vi "PosCentersBackAreaQuadrada.vi"(8 "Robô fora?":bool=TRUE, 9 "geometry":T1, 10 "Defensores":u32[](array[numeric]), 11 "Pos Bola":dbl[](array[numeric]) format="%#_13g") -> (2 "Pos Centers Back":dbl[][](array[numeric]), 3 "Central Position":dbl[](array[numeric]))   [LabVIEW 2017]
uses:
  Core/Field Size.ctl
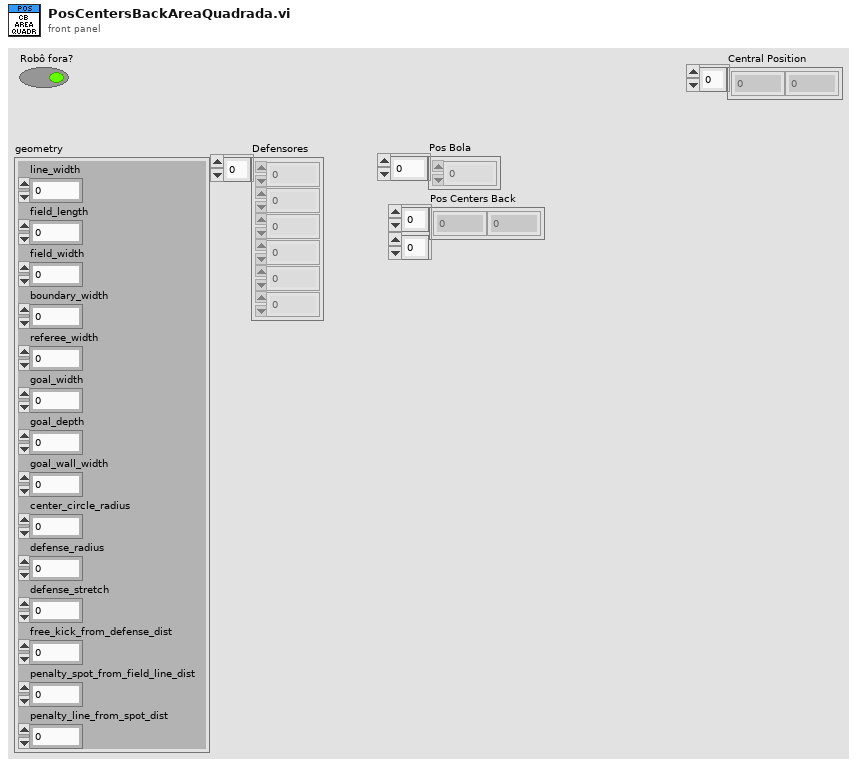
[diagram p1: front panel]
types:
  T1 = typedef "Field Size.ctl" = cluster{"line_width":u32, "field_length":u32, "field_width":u32, "boundary_width":u32, "referee_width":u32, "goal_width":u32, "goal_depth":u32, "goal_wall_width":u32, "center_circle_radius":u32, "defense_radius":u32, "defense_stretch":u32, "free_kick_from_defense_dist":u32, "penalty_spot_from_field_line_dist":u32, "penalty_line_from_spot_dist":u32}
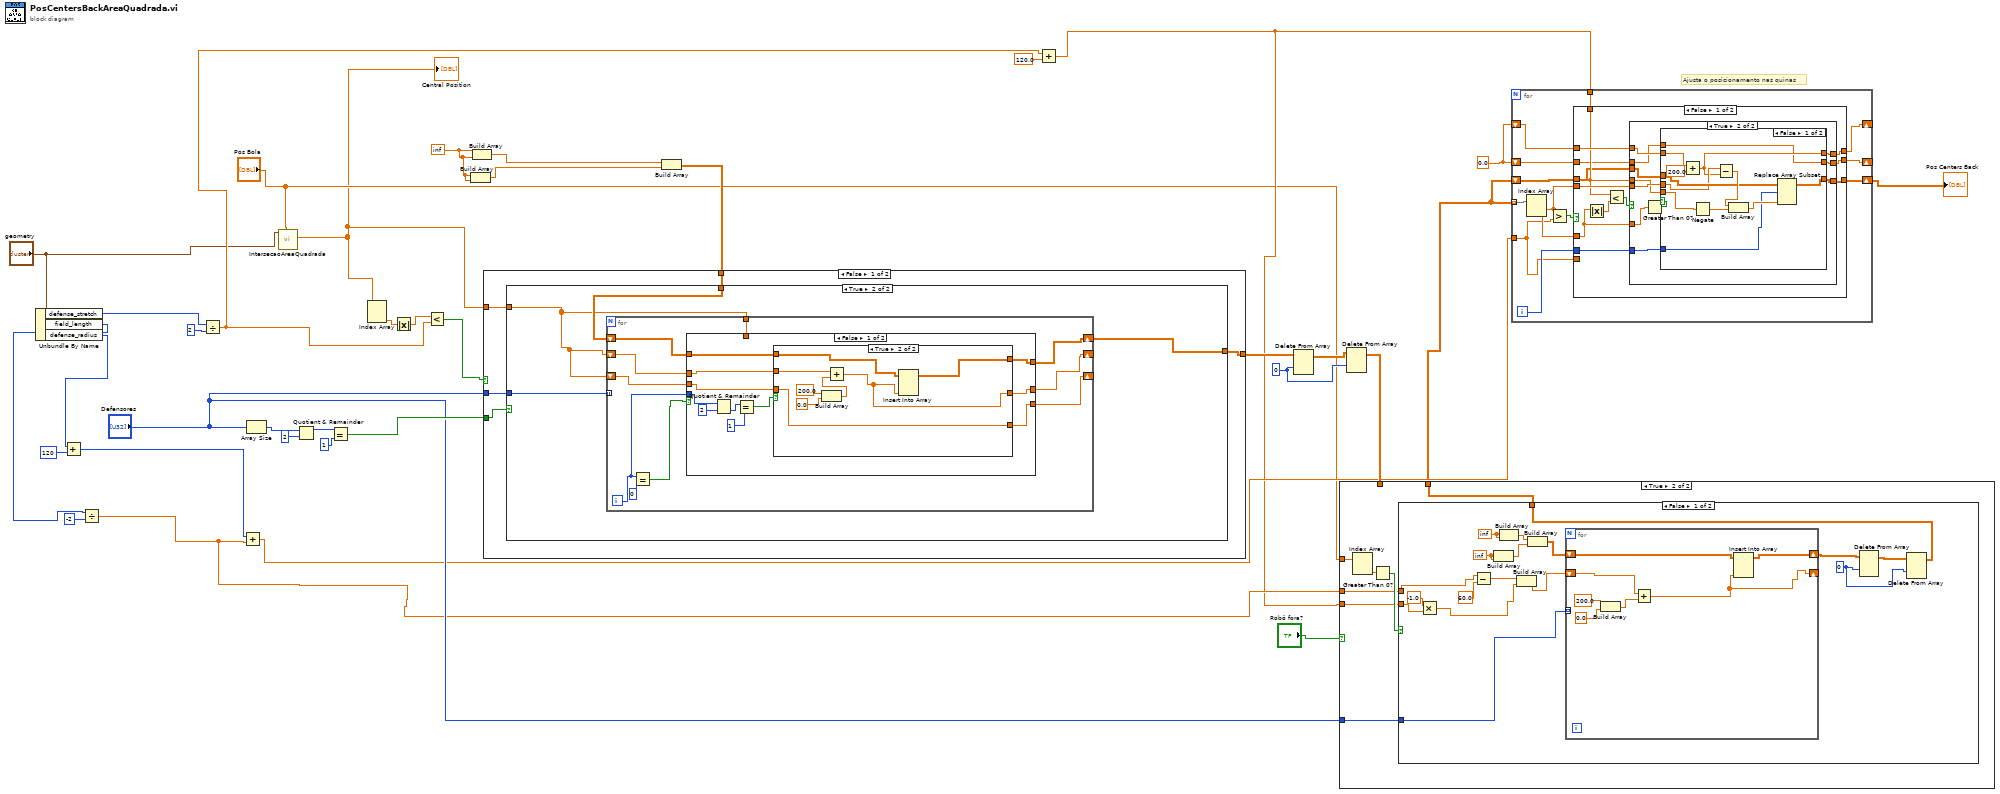
[diagram p0: block diagram]
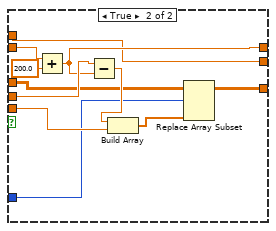
[diagram p3: hidden frame]
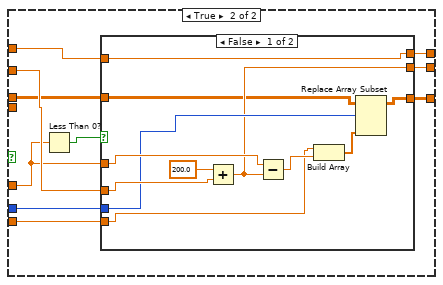
[diagram p4: hidden frame]
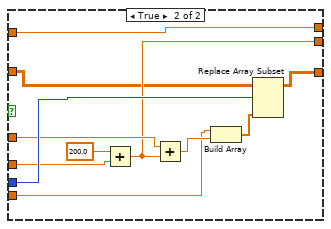
[diagram p5: hidden frame]
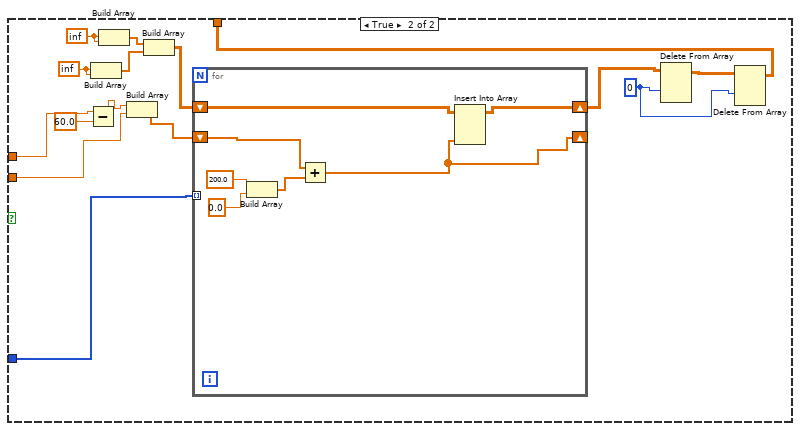
[diagram p7: hidden frame]
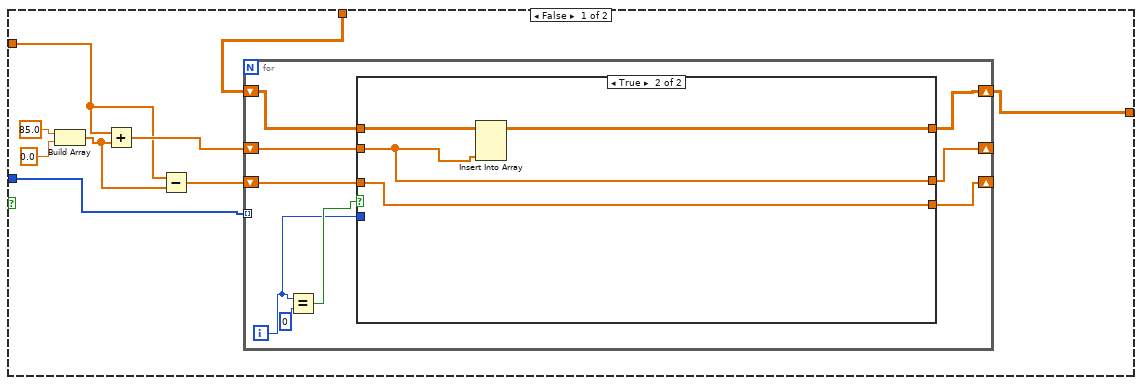
[diagram p8: hidden frame]
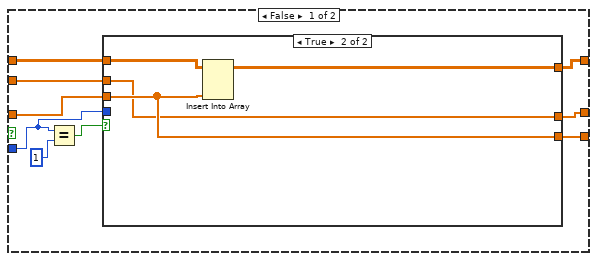
[diagram p9: hidden frame]
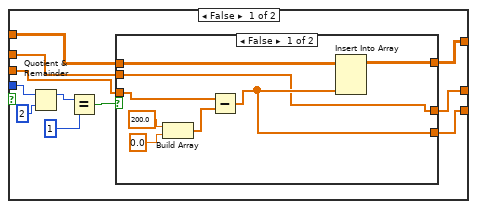
[diagram p10: hidden frame]
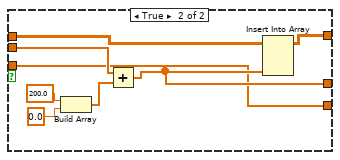
[diagram p11: hidden frame]
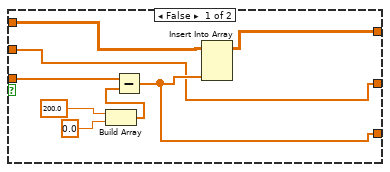
[diagram p12: hidden frame]
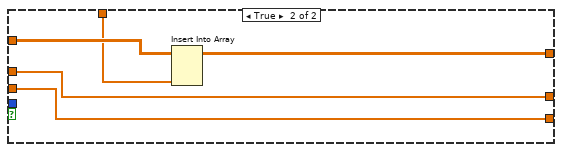
[diagram p13: hidden frame]
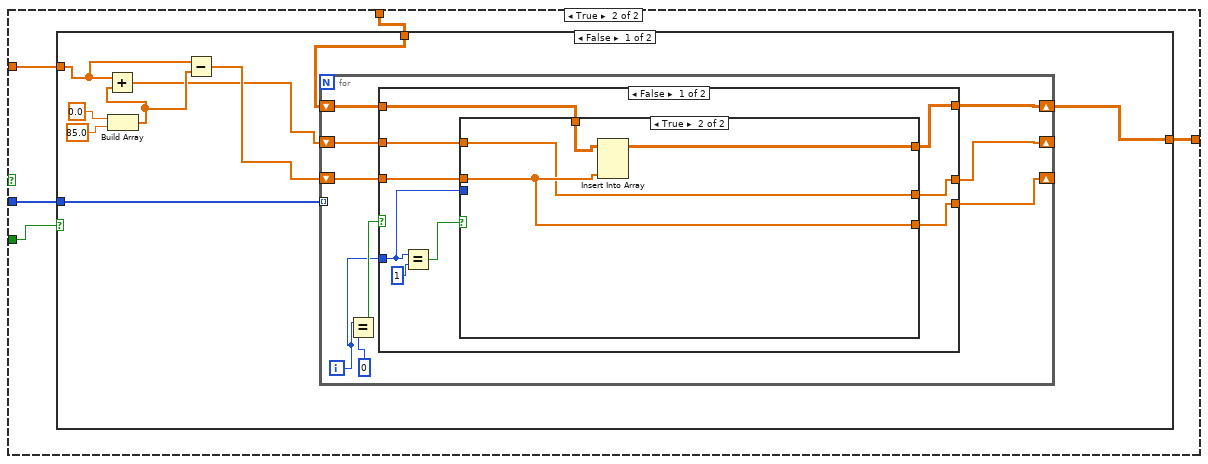
[diagram p14: hidden frame]
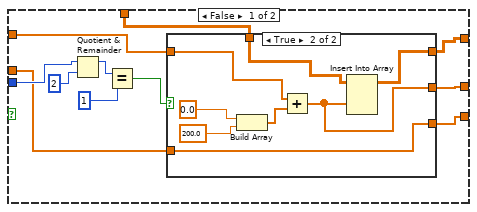
[diagram p15: hidden frame]
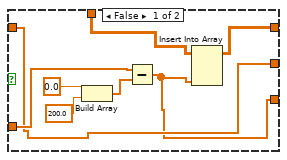
[diagram p16: hidden frame]
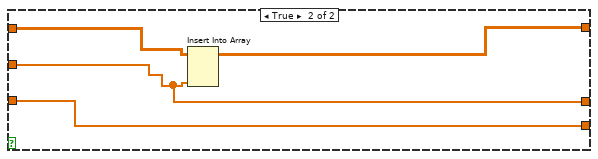
[diagram p17: hidden frame]
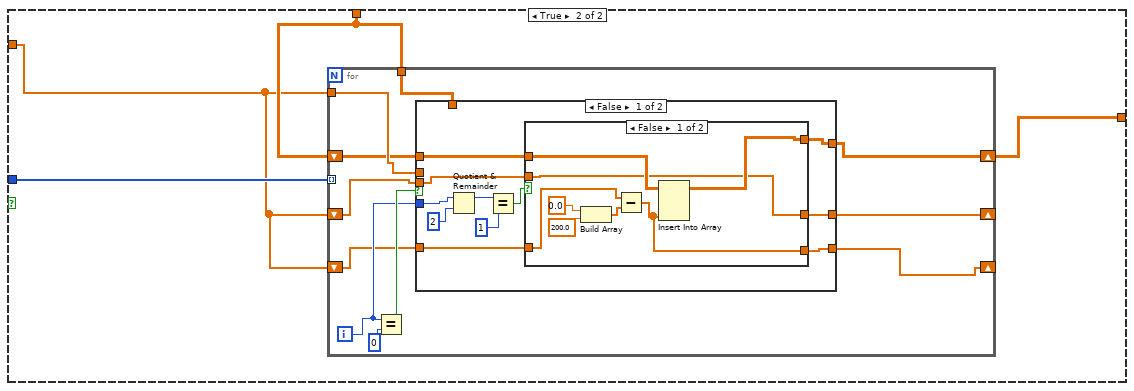
[diagram p18: hidden frame]
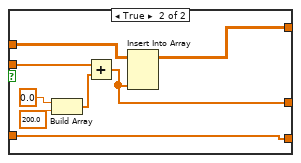
[diagram p19: hidden frame]
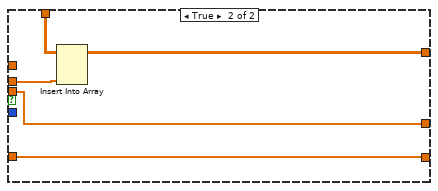
[diagram p20: hidden frame]
diagram:
  w15 = 0.0
  w21 = 0 ("index (row)")
  w27 = inf
  # "Ajusta o posicionamento nas quinas"
  n1 = Unbundle By Name("geometry") -> ("defense_stretch"=w9:u32, "field_length"=w18:u32, "defense_radius"=w11:u32)
  n2 = Add(x=w11, y=u32 120) -> (x+y=w7:u32)
  n3 = Divide(x=w18, y=-2) -> (x/y=w12:dbl)
  n4 = Divide(x=w9, y=u32 2) -> (x/y=w8:dbl)
  n5 = Add(x=w7, y=w12) -> (x+y=w13:dbl)
  n6 = Array Size(array="Defensores") -> (size(s)=w32:i32)
  n7 = call "IntersecaoAreaQuadrada.vi"("Pos entrada"="Pos Bola", "geometry"="geometry") -> ("Pos de Interseção"=w1:dbl[])  [unwired: 8 in, 1 out]
  "Central Position" <- w1
  n8 = Quotient & Remainder(x=w32, y=2) -> (x-y*floor(x/y)=w30:i32)  [unwired: 1 out]
  n9 = Equal?(x=w30, y=1) -> (x = y?=w28:bool)
  n10 = Index Array(array=w1) -> (element #2=w35:dbl)  [unwired: 2 in, 1 out]
  n11 = Absolute Value(x=w35) -> (abs(x)=w34:dbl)
  n12 = Less?(x=w34, y=w8) -> (x < y?=w33:bool)
  n13 = Build Array(w27, w27) -> (w25:dbl[])
  n14 = Build Array(w27, w27) -> (w26:dbl[])
  n15 = Build Array(w26, w25) -> (w24:dbl[][])
  n16 = case shown="False" w33 {
    tunnel: w28 -> [w41 w154]
    tunnel: "Defensores" -> [w40 w153]
    tunnel: w1 -> [w38 w152]
    tunnel: w24 -> [w39 w151]
    tunnel: [w37 w150] -> w23
    frame False {
      n17 = case shown="True" w41 {
        tunnel: w40 -> [w42 w107]
        tunnel: w39 -> [w44 w106]
        tunnel: w38 -> [w47 w105]
        tunnel: [w43 w104] -> w37
        frame False {
          n18 = Build Array(85.0, 0.0) -> (w46:dbl[])
          n19 = Add(x=w47, y=w46) -> (x+y=w48:dbl[])
          n20 = Subtract(x=w47, y=w46) -> (x-y=w45:dbl[])
          n21 = for {
            shift-right: [w54] -> _
            shift-left: w48 -> [w56]
            shift-right: [w53] -> _
            shift-left: w45 -> [w52]
            shift-right: [w55] -> w43
            shift-left: w44 -> [w57]
            tunnel: w42 -> [_] mode=indexing
            i -> [w51]
            n22 = Equal?(x=w51, y=0) -> (x = y?=w58:bool)
            n23 = case shown="True" w58 {
              tunnel: w57 -> [w66 w103]
              tunnel: w56 -> [w62 w101]
              tunnel: [w61 w102] -> w55
              tunnel: [w63 w101] -> w54
              tunnel: [w64 w100] -> w53
              tunnel: w52 -> [w65 w100]
              tunnel: w51 -> [w60 _]
              frame False {
                n24 = Equal?(x=w60, y=1) -> (x = y?=w67:bool)
                n25 = case shown="True" w67 {
                  tunnel: w66 -> [w74 w99]
                  tunnel: w65 -> [w69 w98]
                  tunnel: [w70 w98] -> w64
                  tunnel: [w71 w97] -> w63
                  tunnel: w62 -> [w73 w97]
                  tunnel: [w72 w96] -> w61
                  tunnel: w60 -> [w79 _]
                  frame False {
                    n26 = Quotient & Remainder(x=w79, y=2) -> (x-y*floor(x/y)=w77:i32)  [unwired: 1 out]
                    n27 = Equal?(x=w77, y=1) -> (x = y?=w75:bool)
                    n28 = case shown="False" w75 {
                      tunnel: w74 -> [w86 w95]
                      tunnel: w73 -> [w80 w91]
                      tunnel: [w87 w90] -> w72
                      tunnel: [w80 w89] -> w71
                      tunnel: [w81 w88] -> w70
                      tunnel: w69 -> [w82 w88]
                      frame False {
                        n29 = Build Array(200.0, 0.0) -> (w83:dbl[])
                        n30 = Subtract(x=w82, y=w83) -> (x-y=w81:dbl[])
                        n31 = Insert Into Array(array=w86, new element=w81) -> (w87:dbl[][])  [unwired: 2 in]
                      }
                      frame True {
                        n32 = Build Array(200.0, 0.0) -> (w92:dbl[])
                        n33 = Add(x=w91, y=w92) -> (x+y=w89:dbl[])
                        n34 = Insert Into Array(array=w95, new element=w89) -> (w90:dbl[][])  [unwired: 2 in]
                      }
                    }
                  }
                  frame True {
                    n35 = Insert Into Array(array=w99, new element=w98) -> (w96:dbl[][])  [unwired: 2 in]
                  }
                }
              }
              frame True {
                n36 = Insert Into Array(array=w103, new element=w101) -> (w102:dbl[][])  [unwired: 2 in]
              }
            }
          }
        }
        frame True {
          n37 = for {
            tunnel: w107 -> [_] mode=indexing
            shift-right: [w113] -> w104
            shift-left: w106 -> [w115]
            shift-right: [w111] -> _
            shift-left: w105 -> [w110]
            shift-right: [w109] -> _
            shift-left: w105 -> [w108]
            tunnel: w105 -> [w114]
            i -> [w112]
            n38 = Equal?(x=w112, y=0) -> (x = y?=w116:bool)
            n39 = case shown="False" w116 {
              tunnel: w115 -> [w123 w149]
              tunnel: w114 -> [_ w148]
              tunnel: [w122 w147] -> w113
              tunnel: w112 -> [w128 _]
              tunnel: [w119 w146] -> w111
              tunnel: w110 -> [w124 w146]
              tunnel: [w120 w145] -> w109
              tunnel: w108 -> [w121 w145]
              frame False {
                n40 = Quotient & Remainder(x=w128, y=2) -> (floor(x/y)=w126:i32)  [unwired: 1 out]
                n41 = Equal?(x=w126, y=1) -> (x = y?=w118:bool)
                n42 = case shown="True" w118 {
                  tunnel: w124 -> [w130 w142]
                  tunnel: w123 -> [w133 w140]
                  tunnel: [w132 w139] -> w122
                  tunnel: w121 -> [w134 w138]
                  tunnel: [w131 w138] -> w120
                  tunnel: [w130 w137] -> w119
                  frame False {
                    n43 = Build Array(200.0, 0.0 ("element")) -> (w135:dbl[])
                    n44 = Subtract(x=w134, y=w135) -> (x-y=w131:dbl[])
                    n45 = Insert Into Array(array=w133, new element=w131) -> (w132:dbl[][])  [unwired: 2 in]
                  }
                  frame True {
                    n46 = Build Array(200.0, 0.0) -> (w141:dbl[])
                    n47 = Add(x=w142, y=w141) -> (x+y=w137:dbl[])
                    n48 = Insert Into Array(array=w140, new element=w137) -> (w139:dbl[][])  [unwired: 2 in]
                  }
                }
              }
              frame True {
                n49 = Insert Into Array(array=w149, new element=w148) -> (w147:dbl[][])  [unwired: 2 in]
              }
            }
          }
        }
      }
    }
    frame True {
      n50 = case shown="False" w154 {
        tunnel: w153 -> [w163 w220]
        tunnel: w152 -> [w160 w218]
        tunnel: w151 -> [w158 w219]
        tunnel: [w155 w217] -> w150
        frame False {
          n51 = Build Array(0.0, 85.0) -> (w159:dbl[])
          n52 = Add(x=w160, y=w159) -> (x+y=w156:dbl[])
          n53 = Subtract(x=w160, y=w159) -> (x-y=w157:dbl[])
          n54 = for {
            tunnel: w163 -> [_] mode=indexing
            shift-right: [w164] -> _
            shift-left: w156 -> [w169]
            shift-right: [w168] -> w155
            shift-left: w158 -> [w170]
            shift-right: [w165] -> _
            shift-left: w157 -> [w166]
            i -> [w167]
            n55 = Equal?(x=w167, y=0) -> (x = y?=w171:bool)
            n56 = case shown="False" w171 {
              tunnel: w170 -> [w179 w216]
              tunnel: w169 -> [w174 w213]
              tunnel: [w177 w215] -> w168
              tunnel: w167 -> [w173 _]
              tunnel: w166 -> [w178 w214]
              tunnel: [w176 w214] -> w165
              tunnel: [w175 w213] -> w164
              frame False {
                n57 = Equal?(x=w173, y=1) -> (x = y?=w180:bool)
                n58 = case shown="True" w180 {
                  tunnel: w179 -> [w187 w212]
                  tunnel: w178 -> [w183 w210]
                  tunnel: [w186 w211] -> w177
                  tunnel: [w184 w210] -> w176
                  tunnel: [w185 w209] -> w175
                  tunnel: w174 -> [w188 w209]
                  tunnel: w173 -> [w192 _]
                  frame False {
                    n59 = Quotient & Remainder(x=w192, y=2) -> (x-y*floor(x/y)=w182:i32)  [unwired: 1 out]
                    n60 = Equal?(x=w182, y=1) -> (x = y?=w189:bool)
                    n61 = case shown="True" w189 {
                      tunnel: w188 -> [w194 w205]
                      tunnel: w187 -> [w195 w204]
                      tunnel: [w196 w203] -> w186
                      tunnel: [w194 w202] -> w185
                      tunnel: [w193 w201] -> w184
                      tunnel: w183 -> [w197 w201]
                      frame False {
                        n62 = Build Array(0.0, 200.0) -> (w200:dbl[])
                        n63 = Subtract(x=w197, y=w200) -> (x-y=w193:dbl[])
                        n64 = Insert Into Array(array=w195, new element=w193) -> (w196:dbl[][])  [unwired: 2 in]
                      }
                      frame True {
                        n65 = Build Array(0.0, 200.0) -> (w206:dbl[])
                        n66 = Add(x=w205, y=w206) -> (x+y=w202:dbl[])
                        n67 = Insert Into Array(array=w204, new element=w202) -> (w203:dbl[][])  [unwired: 2 in]
                      }
                    }
                  }
                  frame True {
                    n68 = Insert Into Array(array=w212, new element=w210) -> (w211:dbl[][])  [unwired: 2 in]
                  }
                }
              }
              frame True {
                n69 = Insert Into Array(array=w216, new element=w213) -> (w215:dbl[][])  [unwired: 2 in]
              }
            }
          }
        }
        frame True {
          n70 = for {
            tunnel: w220 -> [_] mode=indexing
            tunnel: w219 -> [w230]
            tunnel: w218 -> [w229]
            shift-right: [w228] -> w217
            shift-left: w219 -> [w225]
            shift-right: [w223] -> _
            shift-left: w218 -> [w224]
            shift-right: [w221] -> _
            shift-left: w218 -> [w222]
            i -> [w226]
            n71 = Equal?(x=w226, y=0) -> (x = y?=w231:bool)
            n72 = case shown="False" w231 {
              tunnel: w230 -> [_ w263]
              tunnel: w229 -> [_ w262]
              tunnel: [w236 w261] -> w228
              tunnel: w226 -> [w242 _]
              tunnel: w225 -> [w237 _]
              tunnel: w224 -> [w235 w260]
              tunnel: [w234 w260] -> w223
              tunnel: w222 -> [w233 w259]
              tunnel: [w232 w259] -> w221
              frame False {
                n73 = Quotient & Remainder(x=w242, y=2) -> (x-y*floor(x/y)=w240:i32)  [unwired: 1 out]
                n74 = Equal?(x=w240, y=1) -> (x = y?=w238:bool)
                n75 = case shown="False" w238 {
                  tunnel: w237 -> [w246 w255]
                  tunnel: [w245 w254] -> w236
                  tunnel: w235 -> [w243 w253]
                  tunnel: [w243 w252] -> w234
                  tunnel: w233 -> [w247 w251]
                  tunnel: [w244 w251] -> w232
                  frame False {
                    n76 = Build Array(0.0, 200.0) -> (w248:dbl[])
                    n77 = Subtract(x=w247, y=w248) -> (x-y=w244:dbl[])
                    n78 = Insert Into Array(array=w246, new element=w244) -> (w245:dbl[][])  [unwired: 2 in]
                  }
                  frame True {
                    n79 = Build Array(0.0, 200.0) -> (w256:dbl[])
                    n80 = Add(x=w253, y=w256) -> (x+y=w252:dbl[])
                    n81 = Insert Into Array(array=w255, new element=w252) -> (w254:dbl[][])  [unwired: 2 in]
                  }
                }
              }
              frame True {
                n82 = Insert Into Array(array=w263, new element=w262) -> (w261:dbl[][])  [unwired: 2 in]
              }
            }
          }
        }
      }
    }
  }
  n83 = Add(x=w8, y=120.0) -> (x+y=w4:dbl)
  n84 = Delete From Array(array=w23, index (row)=w21) -> (array with subset deleted=w22:dbl[][])  [unwired: 2 in, 1 out]
  n85 = Delete From Array(array=w22, index (row)=w21) -> (array with subset deleted=w19:dbl[][])  [unwired: 2 in, 1 out]
  n86 = case shown="True" "Robô fora?" {
    tunnel: "Pos Bola" -> [_ w271]
    tunnel: [w264 w266] -> w6
    tunnel: w19 -> [w264 _]
    tunnel: w12 -> [_ w268]
    tunnel: "Defensores" -> [_ w267]
    tunnel: w4 -> [_ w265]
    frame False {
    }
    frame True {
      n87 = Index Array(array=w271) -> (element #2=w270:dbl)  [unwired: 2 in, 1 out]
      n88 = Greater Than 0?(x=w270) -> (x > 0?=w269:bool)
      n89 = case shown="False" w269 {
        tunnel: w268 -> [w277 w299]
        tunnel: w267 -> [w279 w310]
        tunnel: [w278 w300] -> w266
        tunnel: w265 -> [w273 w296]
        frame False {
          w280 = 0 ("index (row)")
          w285 = inf
          w284 = inf
          n90 = Multiply(x=-1.0, y=w273) -> (x*y=w274:dbl)
          n91 = Subtract(x=w277, y=60.0) -> (x-y=w275:dbl)
          n92 = Build Array(w285, w285) -> (w287:dbl[])
          n93 = Build Array(w284, w284) -> (w286:dbl[])
          n94 = Build Array(w275, w274) -> (w288:dbl[])
          n95 = Build Array(w286, w287) -> (w283:dbl[][])
          n96 = for {
            tunnel: w279 -> [_] mode=indexing
            shift-right: [w290] -> w282
            shift-left: w283 -> [w291]
            shift-right: [w289] -> _
            shift-left: w288 -> [w292]
            n97 = Build Array(200.0, 0.0) -> (w293:dbl[])
            n98 = Add(x=w292, y=w293) -> (x+y=w289:dbl[])
            n99 = Insert Into Array(array=w291, new element=w289) -> (w290:dbl[][])  [unwired: 2 in]
          }
          n100 = Delete From Array(array=w282, index (row)=w280) -> (array with subset deleted=w281:dbl[][])  [unwired: 2 in, 1 out]
          n101 = Delete From Array(array=w281, index (row)=w280) -> (array with subset deleted=w278:dbl[][])  [unwired: 2 in, 1 out]
        }
        frame True {
          w301 = 0 ("index (row)")
          w306 = inf
          w305 = inf
          n102 = Subtract(x=w299, y=60.0) -> (x-y=w297:dbl)
          n103 = Build Array(w306, w306) -> (w308:dbl[])
          n104 = Build Array(w305, w305) -> (w307:dbl[])
          n105 = Build Array(w297, w296) -> (w309:dbl[])
          n106 = Build Array(w307, w308) -> (w304:dbl[][])
          n107 = for {
            tunnel: w310 -> [_] mode=indexing
            shift-right: [w312] -> w303
            shift-left: w304 -> [w313]
            shift-right: [w311] -> _
            shift-left: w309 -> [w314]
            n108 = Build Array(200.0, 0.0) -> (w315:dbl[])
            n109 = Add(x=w314, y=w315) -> (x+y=w311:dbl[])
            n110 = Insert Into Array(array=w313, new element=w311) -> (w312:dbl[][])  [unwired: 2 in]
          }
          n111 = Delete From Array(array=w303, index (row)=w301) -> (array with subset deleted=w302:dbl[][])  [unwired: 2 in, 1 out]
          n112 = Delete From Array(array=w302, index (row)=w301) -> (array with subset deleted=w300:dbl[][])  [unwired: 2 in, 1 out]
        }
      }
    }
  }
  n113 = for {
    tunnel: w6 -> [w328] mode=indexing
    tunnel: w13 -> [w325]
    shift-right: [w324] -> _
    shift-left: w15 -> [w326]
    shift-right: [w322] -> w5
    shift-left: w6 -> [w323]
    tunnel: w4 -> [w321]
    shift-right: [w318] -> _
    shift-left: w15 -> [w320]
    i -> [w327]
    n114 = Index Array(array=w328) -> (element #1=w319:dbl, element #2=w329:dbl)  [unwired: 2 in]
    n115 = Greater?(x=w319, y=w325) -> (0:w330:bool)
    n116 = case shown="False" w330 {
      tunnel: w329 -> [w340 w386]
      tunnel: w327 -> [w335 w388]
      tunnel: w326 -> [w332 w387]
      tunnel: w325 -> [_ w385]
      tunnel: [w331 w384] -> w324
      tunnel: w323 -> [w334 w383]
      tunnel: [w333 w382] -> w322
      tunnel: w321 -> [w336 _]
      tunnel: w320 -> [w339 w380]
      tunnel: w319 -> [w338 _]
      tunnel: [w337 w381] -> w318
      frame False {
        n117 = Absolute Value(x=w340) -> (abs(x)=w342:dbl)
        n118 = Less?(x=w336, y=w342) -> (x < y?=w341:bool)
        n119 = case shown="True" w341 {
          tunnel: w340 -> [_ w356]
          tunnel: w339 -> [w344 w354]
          tunnel: w338 -> [_ w353]
          tunnel: [w344 w352] -> w337
          tunnel: w336 -> [_ w351]
          tunnel: w335 -> [_ w350]
          tunnel: w334 -> [w345 w349]
          tunnel: [w345 w348] -> w333
          tunnel: w332 -> [w343 w347]
          tunnel: [w343 w346] -> w331
          frame False {
          }
          frame True {
            n120 = Greater Than 0?(x=w356) -> (x > 0?=w355:bool)
            n121 = case shown="False" w355 {
              tunnel: w354 -> [w363 w379]
              tunnel: w353 -> [w362 w377]
              tunnel: [w359 w376] -> w352
              tunnel: w351 -> [w360 w374]
              tunnel: w350 -> [w357 w373]
              tunnel: w349 -> [w364 w371]
              tunnel: [w365 w370] -> w348
              tunnel: w347 -> [w358 w369]
              tunnel: [w358 w369] -> w346
              frame False {
                n122 = Add(x=w363, y=200.0) -> (x+y=w359:dbl)
                n123 = Negate(x=w360) -> (-x=w361:dbl)
                n124 = Subtract(x=w362, y=w359) -> (x-y=w367:dbl)
                n125 = Build Array(w367, w361) -> (w366:dbl[])
                n126 = Replace Array Subset(array=w364, new element=w366, index (row)=w357) -> (w365:dbl[][])  [unwired: 1 in]
              }
              frame True {
                n127 = Add(x=w379, y=200.0) -> (x+y=w376:dbl)
                n128 = Subtract(x=w377, y=w376) -> (x-y=w375:dbl)
                n129 = Build Array(w375, w374) -> (w372:dbl[])
                n130 = Replace Array Subset(array=w371, new element=w372, index (row)=w373) -> (w370:dbl[][])  [unwired: 1 in]
              }
            }
          }
        }
      }
      frame True {
        n131 = Less Than 0?(x=w386) -> (x < 0?=w389:bool)
        n132 = case shown="False" w389 {
          tunnel: w388 -> [w396 w411]
          tunnel: w387 -> [w398 w410]
          tunnel: w386 -> [w397 w408]
          tunnel: w385 -> [w395 w405]
          tunnel: [w394 w404] -> w384
          tunnel: w383 -> [w393 w403]
          tunnel: [w392 w402] -> w382
          tunnel: [w391 w401] -> w381
          tunnel: w380 -> [w391 w401]
          frame False {
            n133 = Add(x=200.0, y=w398) -> (x+y=w394:dbl)
            n134 = Subtract(x=w397, y=w394) -> (x-y=w400:dbl)
            n135 = Build Array(w395, w400) -> (w399:dbl[])
            n136 = Replace Array Subset(array=w393, new element=w399, index (row)=w396) -> (w392:dbl[][])  [unwired: 1 in]
          }
          frame True {
            n137 = Add(x=200.0, y=w410) -> (x+y=w404:dbl)
            n138 = Add(x=w408, y=w404) -> (x+y=w407:dbl)
            n139 = Build Array(w405, w407) -> (w406:dbl[])
            n140 = Replace Array Subset(array=w403, new element=w406, index (row)=w411) -> (w402:dbl[][])  [unwired: 1 in]
          }
        }
      }
    }
  }
  "Pos Centers Back" <- w5
